vi "Init_Processing_Image_Settings-1.vi"(1 "BCG Values #2":T2={"Brightness"=128.0, "Contrast"=45.0, "Gamma"=1.0} {"Brightness" min=0 max=255 step=1 format="%.2f"; "Contrast" min=1 max=89 step=1 format="%.2f"; "Gamma" min=0.1 max=10 step=0.01 format="%.2f"}, 2 "BCG Values #1":T2={"Brightness"=128.0, "Contrast"=45.0, "Gamma"=1.0} {"Brightness" min=0 max=255 step=1 format="%.2f"; "Contrast" min=1 max=89 step=1 format="%.2f"; "Gamma" min=0.1 max=10 step=0.01 format="%.2f"}, 3 "Sigma #2":dbl, 4 "Dim #2":u8, 5 "Sigma #1":dbl, 6 "Dim #1":u8) -> (0 "Process Settings":T1)   [LabVIEW 2013]
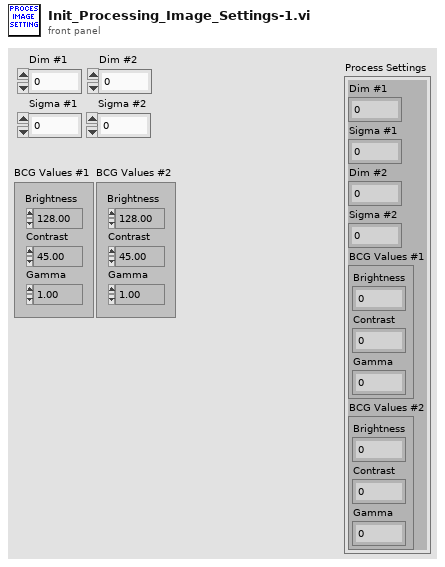
[diagram p1: front panel]
types:
  T1 = cluster{"Dim #1":u8, "Sigma #1":dbl, "Dim #2":u8, "Sigma #2":dbl, "BCG Values #1":cluster{"Brightness":sgl, "Contrast":sgl, "Gamma":sgl}, "BCG Values #2":cluster{"Brightness":sgl, "Contrast":sgl, "Gamma":sgl}}
  T2 = cluster{"Brightness":sgl, "Contrast":sgl, "Gamma":sgl}
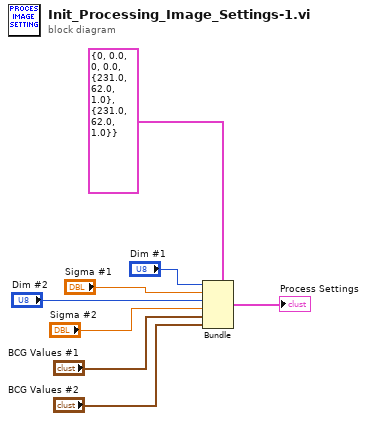
[diagram p0: block diagram]
diagram:
  n1 = Bundle(cluster=T1 {"Dim #1"=0, "Sigma #1"=0.0, "Dim #2"=0, "Sigma #2"=0.0, "BCG Values #1"={"Brightness"=231.0, "Contrast"=62.0, "Gamma"=1.0}, "BCG Values #2"={"Brightness"=231.0, "Contrast"=62.0, "Gamma"=1.0}}, "Dim #1"="Dim #1", "Sigma #1"="Sigma #1", "Dim #2"="Dim #2", "Sigma #2"="Sigma #2", "BCG Values #1"="BCG Values #1", "BCG Values #2"="BCG Values #2") -> (→"Process Settings":T1)
